vi "hmi_shutdown.vi"(7 "hmi_references":T1, 8 "error in (no error)":errorcluster) -> (0 "error out":errorcluster)   [LabVIEW 2015, in "lv-build-interface.lvlib"]
uses:
  lv-build-interface.lvlib
  _controls/hmi_references.ctl
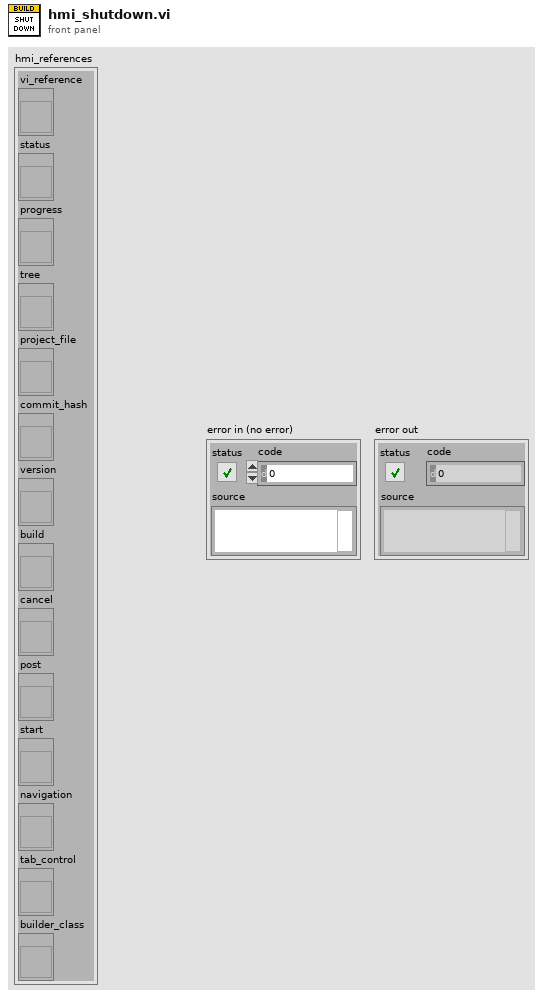
[diagram p1: front panel]
types:
  T1 = typedef "lv-build-interface.lvlib/hmi_references.ctl" = cluster{"vi_reference":refnum<vi>, "status":refnum<vi>, "progress":refnum<vi>, "tree":refnum<vi>, "project_file":refnum<vi>, "commit_hash":refnum<vi>, "version":refnum<vi>, "build":refnum<vi>, "cancel":refnum<vi>, "post":refnum<vi>, "start":refnum<vi>, "navigation":refnum<vi>, "tab_control":refnum<vi>, "builder_class":refnum<vi>}
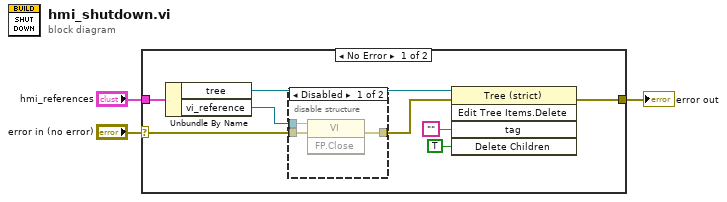
[diagram p0: block diagram]
diagram:
  n1 = case shown="No Error" "error in (no error)" {
    selector: "error in (no error)" -> [w9 w16]
    tunnel: [w4 w16] -> w2
    tunnel: "hmi_references" -> [w10 _]
    frame No Error {
      n2 = Unbundle By Name(w10) -> ("tree"=w6:refnum<vi>, "vi_reference"=w11:refnum<vi>)
      n3 = disable-structure shown="Disabled" {
        disable-tunnel: w11 -> [w14 _]
        disable-tunnel: w9 -> [w13 w15]
        disable-tunnel: [w12 w15] -> w5
        frame Disabled {
          n4 = invoke class="VI" method="FP.Close"(reference=w14, error in=w13) -> (error out=w12:errorcluster)  [unwired: 1 in, 2 out]
        }
        frame Enabled {
        }
      }
      n5 = invoke class="Tree (strict)" method="Edit Tree Items.Delete"(reference=w6, error in=w5, "tag"="", "Delete Children"=TRUE ("Delete Children?")) -> (error out=w4:errorcluster)  [unwired: 1 in, 4 out]
    }
    frame Error {
    }
  }
  "error out" <- w2
